vi "2D Array (Random[0,N-1]).vi"(1 "Rows":u64, 3 "Cols":u64, 6 "Dimension":u64) -> (15 "output array":u64[][](array[numeric]))   [LabVIEW 2014]
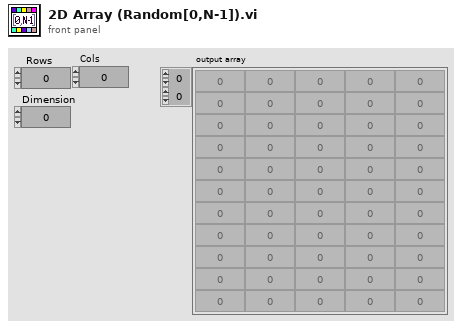
[diagram p1: front panel]
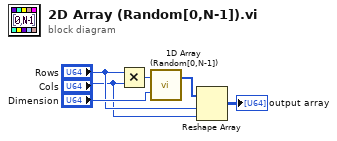
[diagram p0: block diagram]
diagram:
  n1 = Multiply(x="Rows", y="Cols") -> (x*y=w6:u64)
  n2 = call "1D Array (Random[0,N-1]).vi"("Length"=w6, "Dimension"="Dimension") -> ("Array"=w4:u64[])  [unwired: 17 in]
  n3 = Reshape Array(w4, "Rows", "Cols") -> (→"output array":u64[][])
